vi "Read ActorConfiguration.vi"(11 "Template in":refnum<class "Template.lvclass">) -> (3 "ActorConfiguration":T1={"GlobalConfiguration"={"DeviceFamily"="", "WriteData"=FALSE, "BufferSize_samples"=-1, "SyncDevice"=FALSE, "ExecuteInterruptRoutine"=FALSE, "InterruptRoutineTimeout_ms"=-1}, "DeviceConfiguration"={"DeviceSpecificName"="MIPI_Camera", "HardwareReference"="PXIe-Slot2", "UsedResources"=[{"ResourceLocation"="FrontFacing", "ResourceData"=variant(string "Use this Variant to store your specific resource data.\nThis will be read from and written to with the JSON parsing API.\nIn the child implementation you can use the acessors provided to convert from the specific cluster to your own device's implementation")}]}})   [LabVIEW 2020, in "Template.lvlib" / "Template.lvclass"]
doc: "Returns the actor configuration cluster"
uses:
  Template.lvclass
  typedefs/actor configuration.ctl
  typedefs/shared actor configuration.ctl
  typedefs/resource config/device configuration cluster.ctl
  typedefs/resource config/single resource cluster.ctl
  Template.lvclass/Template.ctl
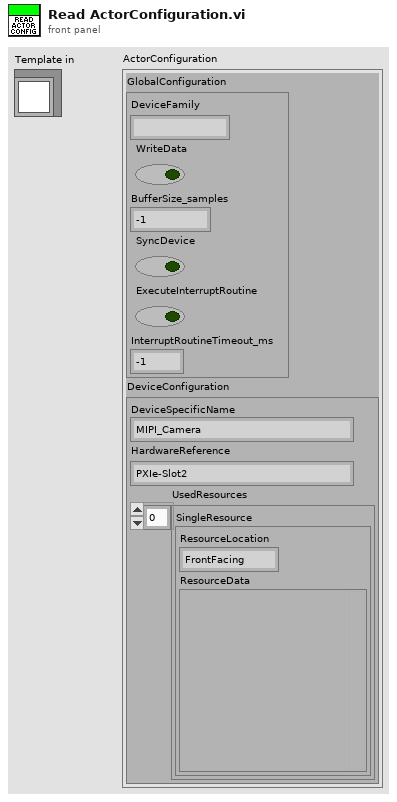
[diagram p1: front panel]
types:
  T1 = typedef "Template.lvlib/Template.lvclass/actor configuration.ctl" = cluster{"GlobalConfiguration":T2, "DeviceConfiguration":T3}
  T2 = typedef "Template.lvlib/Template.lvclass/shared actor configuration.ctl" = cluster{"DeviceFamily":string, "WriteData":bool, "BufferSize_samples":i32, "SyncDevice":bool, "ExecuteInterruptRoutine":bool, "InterruptRoutineTimeout_ms":i32}
  T3 = typedef "Template.lvlib/Template.lvclass/device configuration cluster.ctl" = cluster{"DeviceSpecificName":string, "HardwareReference":string, "UsedResources":T4[]}
  T4 = typedef "Template.lvlib/Template.lvclass/single resource cluster.ctl" = cluster{"ResourceLocation":string, "ResourceData":variant}
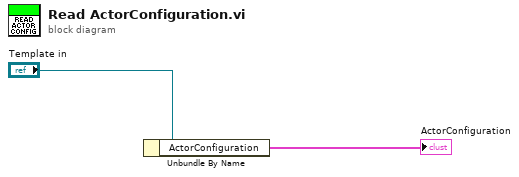
[diagram p0: block diagram]
diagram:
  n1 = Unbundle By Name("Template in") -> ("ActorConfiguration"=→"ActorConfiguration":T1)
